vi "Vision Research Phantom Series PhCon PhGetDllsLogOption.vi"(0 "Value":u32=1, 5 "Error In (no error)":errorcluster) -> (19 "Error Out":errorcluster)   [LabVIEW 2013, in "VRI.lvlib"]
doc: "PhCon.dll\n\nPhGetDllsLogOption\nHRESULT PhGetDllsLogOption(UINT SelectCode, PUINT pValue);\n\nParameters Description\nSelectCode Select the module to get the log options. Use the constants\n defined in PhCon.h:\n GDLO_PHANTOM\n GDLO_PHCON\n GDLO_PHINT\n GDLO_PHFILE\n GDLO_PHSIG\n GDLO_PHSIGV\n GDLO_TORAM\n to select a certain module or option.\npValue Pointer to an unsigned integer that will receive the value of\n the log option for the module or option selected in the first\n parameter.\nReturn HRESULT (0 = Ok)\nComments Call this function to find the current settings for the log \n options on the computer you run your application. These\n settings will be common to all applications that call the \n Phantom libraries and will be persistent between the starts\n of the applications."
uses:
  VRI.lvlib
  _Type Defs/PhCon GDLO.ctl
  Phantom DLLs/PhCon.dll
panel:
  in  "SelectCode":T1=200 items=["GDLO_PHANTOM"=200, "GDLO_PHCON"=201, "GDLO_PHINT"=202, "GDLO_PHFILE"=203, "GDLO_PHSIG"=204, "GDLO_PHSIGV"=205, "GDLO_TORAM"=206]
  # "For instructions on the use of this VI, press Ctrl+H to display the help window and move the mouse over the icon, controls, and indicators"
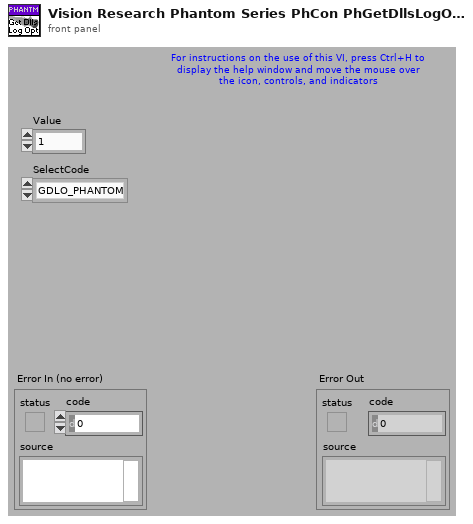
[diagram p1: front panel]
types:
  T1 = typedef "VRI.lvlib/PhCon GDLO.ctl" = u16
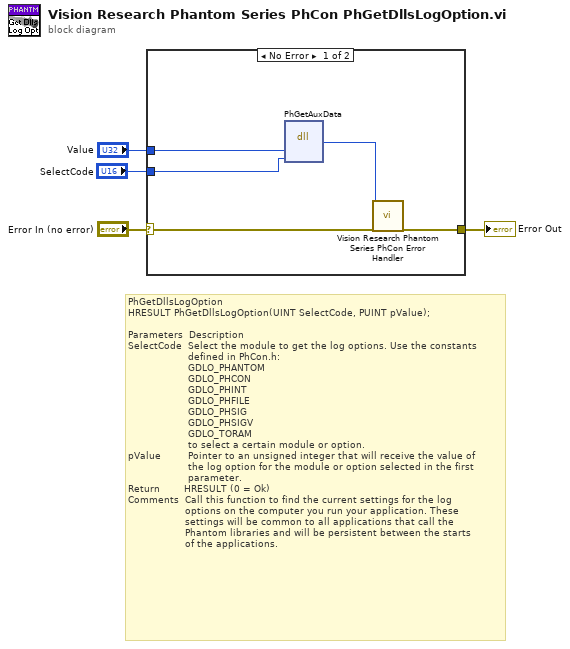
[diagram p0: block diagram]
diagram:
  # "PhGetDllsLogOption\nHRESULT PhGetDllsLogOption(UINT SelectCode, PUINT pValue);\n\nParameters  Description\nSelectCode  Select the module to get the log options. Use the constants\n                    defined in PhCon.h:\n                    GDLO_PHANTOM\n                    GDLO_PHCON\n                    GDLO_PHINT\n                    GDLO_PHFILE\n                    GDLO_PHSIG\n                    GDLO_PHSIGV\n                    GDLO_TORAM\n                    to select a certain module or option.\npValue         Pointer to an unsigned integer that will receive the value of\n                    the log option for the module or option selected in the first\n                    parameter.\nReturn        HRESULT (0 = Ok)\nComments  Call this function to find the current settings for the log \n                   options on the computer you run your application. These\n                   settings will be common to all applications that call the \n                   Phantom libraries and will be persistent between the starts\n                   of the applications."
  n1 = case shown="No Error" "Error In (no error)" {
    selector: "Error In (no error)" -> [w9 w10]
    tunnel: [w8 w10] -> w3
    tunnel: "Value" -> [w7 _]
    tunnel: "SelectCode" -> [w6 _]
    frame No Error {
      n2 = dll-call lib="C:/Projects/SDK/32-bit/Vision Research Phantom Series Labview Driver/Phantom DLLs/PhCon.dll" fn="PhGetAuxData"("SelectCode"=w7, "pValue"=w6) -> ("HRESULT"=w5:i32)  [unwired: 4 in, 3 out]
      n3 = call "Vision Research Phantom Series PhCon Error Handler.vi"("ErrNo"=w5, "Error In (no error)"=w9) -> ("Error Out"=w8:errorcluster)  [unwired: 17 out]
    }
    frame Error {
    }
  }
  "Error Out" <- w3
